vi "dispense status.vi"(11 "dispense status data IN":T1) -> (1 "dispense run off":bool, 2 "dispense run on":bool, 3 "dispense status data OUT":T1)   [LabVIEW 2016]
uses:
  dispense status data.ctl
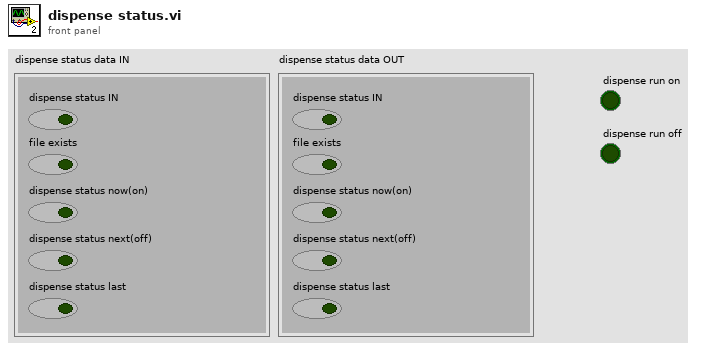
[diagram p1: front panel]
types:
  T1 = typedef "dispense status data.ctl" = cluster{"file exists":bool, "dispense status now(on)":bool, "dispense status next(off)":bool, "dispense status IN":bool, "dispense status last":bool}
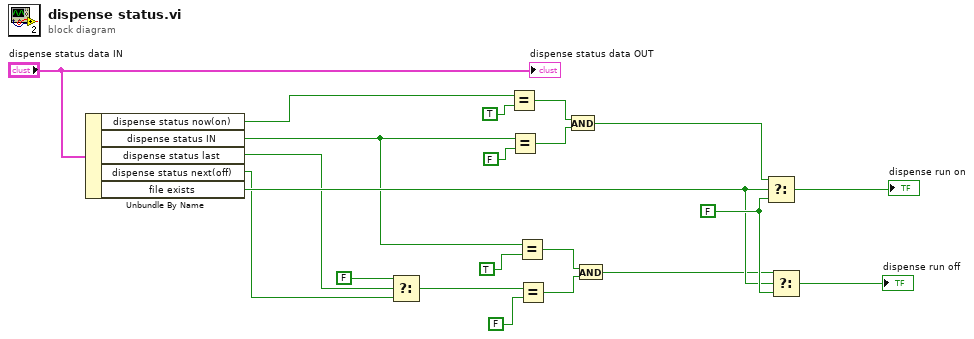
[diagram p0: block diagram]
diagram:
  w9 = FALSE
  n1 = Unbundle By Name("dispense status data IN") -> ("dispense status now(on)"=w19:bool, "dispense status IN"=w1:bool, "dispense status last"=w7:bool, "dispense status next(off)"=w6:bool, "file exists"=w8:bool)
  n2 = Select(t=FALSE, s=w7, f=w6) -> (s? t:f=w5:bool)
  n3 = Equal?(x=w19, y=TRUE) -> (x = y?=w12:bool)
  n4 = Equal?(x=w1, y=FALSE) -> (x = y?=w11:bool)
  n5 = Equal?(x=w1, y=TRUE) -> (x = y?=w17:bool)
  n6 = Equal?(x=w5, y=FALSE) -> (x = y?=w18:bool)
  n7 = And(x=w12, y=w11) -> (x .and. y?=w2:bool)
  n8 = And(x=w17, y=w18) -> (x .and. y?=w4:bool)
  n9 = Select(t=w2, s=w8, f=w9) -> (s? t:f=→"dispense run on":bool)
  n10 = Select(t=w4, s=w8, f=w9) -> (s? t:f=→"dispense run off":bool)
  "dispense status data OUT" <- "dispense status data IN"
